vi "Mark10.vi"(0 "Requested Load":dbl, 1 "Data In":T1={"Message"="", "Homed?"=FALSE, "NextState"=enum."Timeout", "G.Load"=0.0, "G.Position"=0.0, "Load#"=0, "[G.Loads]"=[], "[TotalLoads]"=[], "[Errors]"=[], "ZeroWait"=0, "Results"=[], "DwellWait"=FALSE, "Test Result"=FALSE, "[CondyleLoads]"=[], "[Max]"=[], "[Min]"=[], "Valid String?"=FALSE, "ScanTime"=timestamp(0 s since 1904-01-01), "ScannedString"="", "LabelDevID"=0, "MfgDate"=timestamp(0 s since 1904-01-01), "[EEPROM Cmds]"=[], "[CalData]"=[], "[A/Ds]"=[], "[A/Dmax]"=[], "[A/Dmin]"=[], "BattMax"=0.0, "BattMin"=0.0, "DwellTime"=2000, "PendingDeviceType"="", "Zero G.load"=0.0, "GAINC Value"="", "Programming Step"=enum."Load EEPROM", "Front Panel Program?"=FALSE, "Final Program?"=FALSE, "PCB Score"=100, "AssyScore"=100, "Pass/Fail #"="", "Result String"="", "Programming Mode"=enum."Initial Program", "Angle Test Step"=enum."Initialize", "Accel Values"=[], "Shutdown Counter"=0, "V1"=0, "V2"=0, "V3"=0, "V4"=0, "EEPROM Data"=[], "Counter"=0, "Page#"=0, "Timer"=timestamp(0 s since 1904-01-01), "Use Mark10?"=FALSE, "Eng-Result#"=0, "DUT Serial #"=0, "Scroll Message?"=FALSE, "Clear Message"=FALSE, "Batt Test Step "=enum."Initialize", "RXTX Window Found?"=FALSE, "Shutdown First Call?"=FALSE, "A2 Delay (msec)"=500, "Support Script"={"Script #"="", "Script Revision"="", "[OEMs]"=[], "[[DeviceTypes]]"=[], "[[DeviceTypesVals]]"=[], "[[List of Errors]]"=[], "Default GAINC"="", "[[ASICtrims]]"=[], "ID For Echo"="", "Condyle A CalFactor"=100, "Condyle B CalFactor"=100, "[OEMs Prefix]"=[], "Packet ID 18"="", "[[Force Table Load Test]]"=[], "[[Force Table AccurTest]]"=[]}, "Serial Table"={"Serial File Path"=path "", "[[Serial Lookup Table]]"=[], "Serial Device Info"=[], "Valid Serial?"=FALSE}, "Target Information"={"Target Brand"="", "Target DeviceType"="", "Target Serial#"=100, "Target Lot#"=0, "Target DevID"=0, "Target Channel"=5}, "Operator"="", "COM Port"="", "Config Path"=path "", "Tx Array"=[], "DUT Parameters"={"Channel"=0, "DeviceID"=0, "Script Rev"=0, "Month"=0, "Day"=0, "Year"=0, "Lot#"=0, "V1"=0, "V2"=0, "V3"=0, "V4"=0, "MFG"=0, "Cal FactorA 10"=0, "Cal FactorB 10  "=0, "Cal FactorA 16"=0, "Cal FactorB 16"=0, "ASICtrim"=[], "TmpChan"=0, "GAINC"="", "Brand"="", "Device"="", "Serial #"=0, "Batt310"=0, "Batt 280"=0}, "FTS Main?"=FALSE, "Loading"={"[Forces]"=[], "[Dwell]"=[], "Loading Step"=enum."Initialize Test"}, "Software Version"="", "Correction Factor"="", "Second Load Test"=FALSE, "Acc Loads"=[], "Mark10 Config"={"H2S%"=[80.0, 85.0, 90.0, 95.0, 100.0], "H2S Speed"=[12.0, 8.0, 6.0, 4.0, 2.0], "H to S"=2.0, "Home Speed"=1.0, "LoadWin"=0.0, "Load Speed"=0.0, "PID"={"Kp"=0.04, "Kd"=0.005001, "Ki"=2.9999999999999923e-05}}, "Channels"={"Transceiver Ch"=5, "Operating Ch"=5, "Start Ch"=0}, "Channel EEPROM"=[], "Load Notes"=[], "Engr Log?"=FALSE, "Time"=[], "Program Retry"=FALSE, "Operator Channel"="", "Target Channel "="", "New Data Program"=FALSE, "NFHU Pass?"=FALSE, "Cycle Number"=0, "Cal Cycle#"=0, "[Avg G.Loads] "=[], "[Avg A/Ds] "=[], "Cal Retry?"=FALSE, "[Total A/Ds]  "=[], "Cycle Num LA"=0, "LA Cycle# "=0, "Shim Num"=0, "Shim#  "=0, "Angle Test?"=FALSE} {"Mark10 Config"."PID"."Ki" min=0.0 max=200.0 format="%.6f"; "Mark10 Config"."PID"."Kd" min=0.0 max=200.0 format="%.6f"; "Mark10 Config"."PID"."Kp" min=0.0 max=200.0 format="%.6f"; "DUT Parameters"."ASICtrim" format="%02x"}, 2 "Stop?":bool, 3 "Requested Position":dbl, 4 "Accuracy \nTest?":bool, 5 "error in (no error)":errorcluster, 9 "Action":T16=enum."Stop Motor") -> (10 "Flags":T15, 14 "Live Load":dbl, 16 "Live Position":dbl, 17 "Done?":bool, 19 "error out":errorcluster)   [LabVIEW 2015]
uses:
  Controls/Mark10 states.ctl
  Controls/LocalVars.ctl
  Controls/Gen2 FT states.ctl
  Controls/Iniial Device Programming.ctl
  SubVI/ProgramStageControl.ctl
  Controls/Batt Cap Steps.ctl
  Controls/Support Script.ctl
  Controls/Serial Table.ctl
  Controls/Device Information.ctl
  Controls/InfoPacket.ctl
  Controls/Loading.ctl
  Controls/Load Step.ctl
  Controls/Mark10 Config.ctl
  Controls/PID parameters.ctl
  Controls/Channels.ctl
  Controls/Mark10.ctl
  Controls/Mark10 Comm states.ctl
panel:
  in  "Speed":dbl
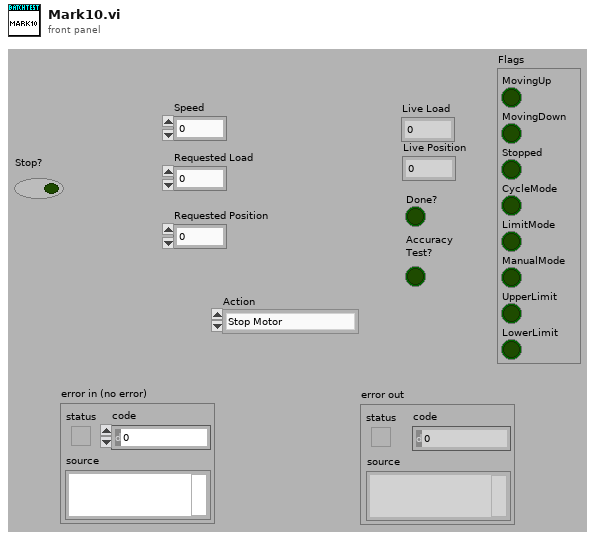
[diagram p1: front panel]
types:
  T1 = typedef "LocalVars.ctl" = cluster{"Message":string, "Homed?":bool, "NextState":T2, "G.Load":dbl, "G.Position":dbl, "Load#":i32, "[G.Loads]":dbl[], "[TotalLoads]":dbl[], "[Errors]":dbl[][], "ZeroWait":u32, "Results":dbl[], "DwellWait":bool, "Test Result":bool, "[CondyleLoads]":dbl[][], "[Max]":dbl[], "[Min]":dbl[], "Valid String?":bool, "ScanTime":timestamp, "ScannedString":string, "LabelDevID":u32, "MfgDate":timestamp, "[EEPROM Cmds]":u8[][], "[CalData]":u8[][], "[A/Ds]":dbl[][], "[A/Dmax]":dbl[], "[A/Dmin]":dbl[], "BattMax":dbl, "BattMin":dbl, "DwellTime":i32, "PendingDeviceType":string, "Zero G.load":dbl, "GAINC Value":string, "Programming Step":T3, "Front Panel Program?":bool, "Final Program?":bool, "PCB Score":i32, "AssyScore":i32, "Pass/Fail #":string, "Result String":string, "Programming Mode":T4, "Angle Test Step":enum16{"Initialize", "Get X", "Get Y", "Get Z", "Next Test"}, "Accel Values":dbl[][], "Shutdown Counter":u32, "V1":i32, "V2":i32, "V3":i32, "V4":i32, "EEPROM Data":i32[][], "Counter":i32, "Page#":i32, "Timer":timestamp, "Use Mark10?":bool, "Eng-Result#":u32, "DUT Serial #":i32, "Scroll Message?":bool, "Clear Message":bool, "Batt Test Step ":T5, "RXTX Window Found?":bool, "Shutdown First Call?":bool, "A2 Delay (msec)":i16, "Support Script":T6, "Serial Table":T7, "Target Information":T8, "Operator":string, "COM Port":string, "Config Path":path, "Tx Array":u8[], "DUT Parameters":T9, "FTS Main?":bool, "Loading":T10, "Software Version":string, "Correction Factor":string, "Second Load Test":bool, "Acc Loads":dbl[][], "Mark10 Config":T12, "Channels":T14, "Channel EEPROM":i32[][], "Load Notes":string[], "Engr Log?":bool, "Time":timestamp[], "Program Retry":bool, "Operator Channel":string, "Target Channel ":string, "New Data Program":bool, "NFHU Pass?":bool, "Cycle Number":i32, "Cal Cycle#":i32, "[Avg G.Loads] ":dbl[], "[Avg A/Ds] ":dbl[][], "Cal Retry?":bool, "[Total A/Ds]  ":dbl[][], "Cycle Num LA":i32, "LA Cycle# ":i32, "Shim Num":i32, "Shim#  ":i32, "Angle Test?":bool}
  T2 = typedef "Gen2 FT states.ctl" = enum16{"---------SETUP-------", "Initialization", "Read Support Data", "Initialize Mark-10", "Initialize Transceiver", "------UTILITIES------", "Change DUT Channel", "Find RxTx Window", "Reset Device", "Scan Channels", "Read Serial Lookup", "Shutdown Device", "ESTOP", "--------USER---------", "Timeout", "-----PROGRAM-----", "Program Device", "------MARK10--------", "Go Home", "MoveUp", "MoveDown", "Goto Load", "Goto Position", "Stop Motor", "---------TESTS--------", "Start Test", "Angle Test", "Load Test", "Load Accuracy Test", "Battery Test", "------RESULTS-------", "End Test", "Display Result", "--------EXIT--------", "Exit"}
  T3 = typedef "Iniial Device Programming.ctl" = enum16{"Load EEPROM", "Send First A1", "Send EEPROM", "Send A1", "Check EEPROM Echo", "Verify transmission", "Programming Successful", "Programming Failed"}
  T4 = typedef "ProgramStageControl.ctl" = enum16{"Initial Program", "GainC", "Scales"}
  T5 = typedef "Batt Cap Steps.ctl" = enum16{"Initialize", "Collect 2.8 Volts", "Collect 3.1 Volts", "Check Results"}
  T6 = typedef "Support Script.ctl" = cluster{"Script #":string, "Script Revision":string, "[OEMs]":string[], "[[DeviceTypes]]":string[][], "[[DeviceTypesVals]]":u16[][], "[[List of Errors]]":string[][], "Default GAINC":string, "[[ASICtrims]]":u8[][], "ID For Echo":string, "Condyle A CalFactor":i32, "Condyle B CalFactor":i32, "[OEMs Prefix]":string[], "Packet ID 18":string, "[[Force Table Load Test]]":dbl[][], "[[Force Table AccurTest]]":dbl[][]}
  T7 = typedef "Serial Table.ctl" = cluster{"Serial File Path":path, "[[Serial Lookup Table]]":string[][], "Serial Device Info":string[], "Valid Serial?":bool}
  T8 = typedef "Device Information.ctl" = cluster{"Target Brand":string, "Target DeviceType":string, "Target Serial#":i32, "Target Lot#":u32, "Target DevID":u32, "Target Channel":u8}
  T9 = typedef "InfoPacket.ctl" = cluster{"Channel":u8, "DeviceID":u32, "Script Rev":u8, "Month":u8, "Day":u8, "Year":u8, "Lot#":u32, "V1":u16, "V2":u16, "V3":u16, "V4":u16, "MFG":u8, "Cal FactorA 10":u8, "Cal FactorB 10  ":u8, "Cal FactorA 16":u8, "Cal FactorB 16":u8, "ASICtrim":u8[], "TmpChan":u8, "GAINC":string, "Brand":string, "Device":string, "Serial #":u64, "Batt310":u16, "Batt 280":u16}
  T10 = typedef "Loading.ctl" = cluster{"[Forces]":dbl[], "[Dwell]":dbl[], "Loading Step":T11}
  T11 = typedef "Load Step.ctl" = enum16{"Initialize Test", "Go Home", "Detect Dev Surface", "Wait to zero Device", "Zero Device", "Do Test", "Test Result"}
  T12 = typedef "Mark10 Config.ctl" = cluster{"H2S%":dbl[], "H2S Speed":dbl[], "H to S":dbl, "Home Speed":dbl, "LoadWin":dbl, "Load Speed":dbl, "PID":T13}
  T13 = typedef "PID parameters.ctl" = cluster{"Kp":dbl, "Kd":dbl, "Ki":dbl}
  T14 = typedef "Channels.ctl" = cluster{"Transceiver Ch":u8, "Operating Ch":u8, "Start Ch":u8}
  T15 = cluster{"MovingUp":bool, "MovingDown":bool, "Stopped":bool, "CycleMode":bool, "LimitMode":bool, "ManualMode":bool, "UpperLimit":bool, "LowerLimit":bool}
  T16 = typedef "Mark10 states.ctl" = enum16{"Initialize", "Go Home", "Move Up", "Move Down", "Stop @ Load", "Read Status", "Goto Position", "Goto Device Surface", "Stop Motor", "Shutdown", "Exit"}
  T17 = typedef "Mark10 Comm states.ctl" = enum16{"Open Session", "Get Reference", "Write Data", "Read Data", "Close Session"}
  T18 = typedef "Mark10.ctl" = cluster{"Mark10 Ref":refnum<visa-resource-name>, "Counter":i32, "MotorSpeed":dbl, "LastSpeed":dbl, "Live Load":dbl, "Live Position":dbl, "Stage":i32, "Speeds":dbl[], "DevFound?":bool, "DevPosition":dbl, "Flags":cluster{"MovingUp":bool, "MovingDown":bool, "Stopped":bool, "CycleMode":bool, "LimitMode":bool, "ManualMode":bool, "UpperLimit":bool, "LowerLimit":bool}, "Stopped?":bool, "ofPass":i32, "LastDrive":dbl, "Mark10 Config":T12}
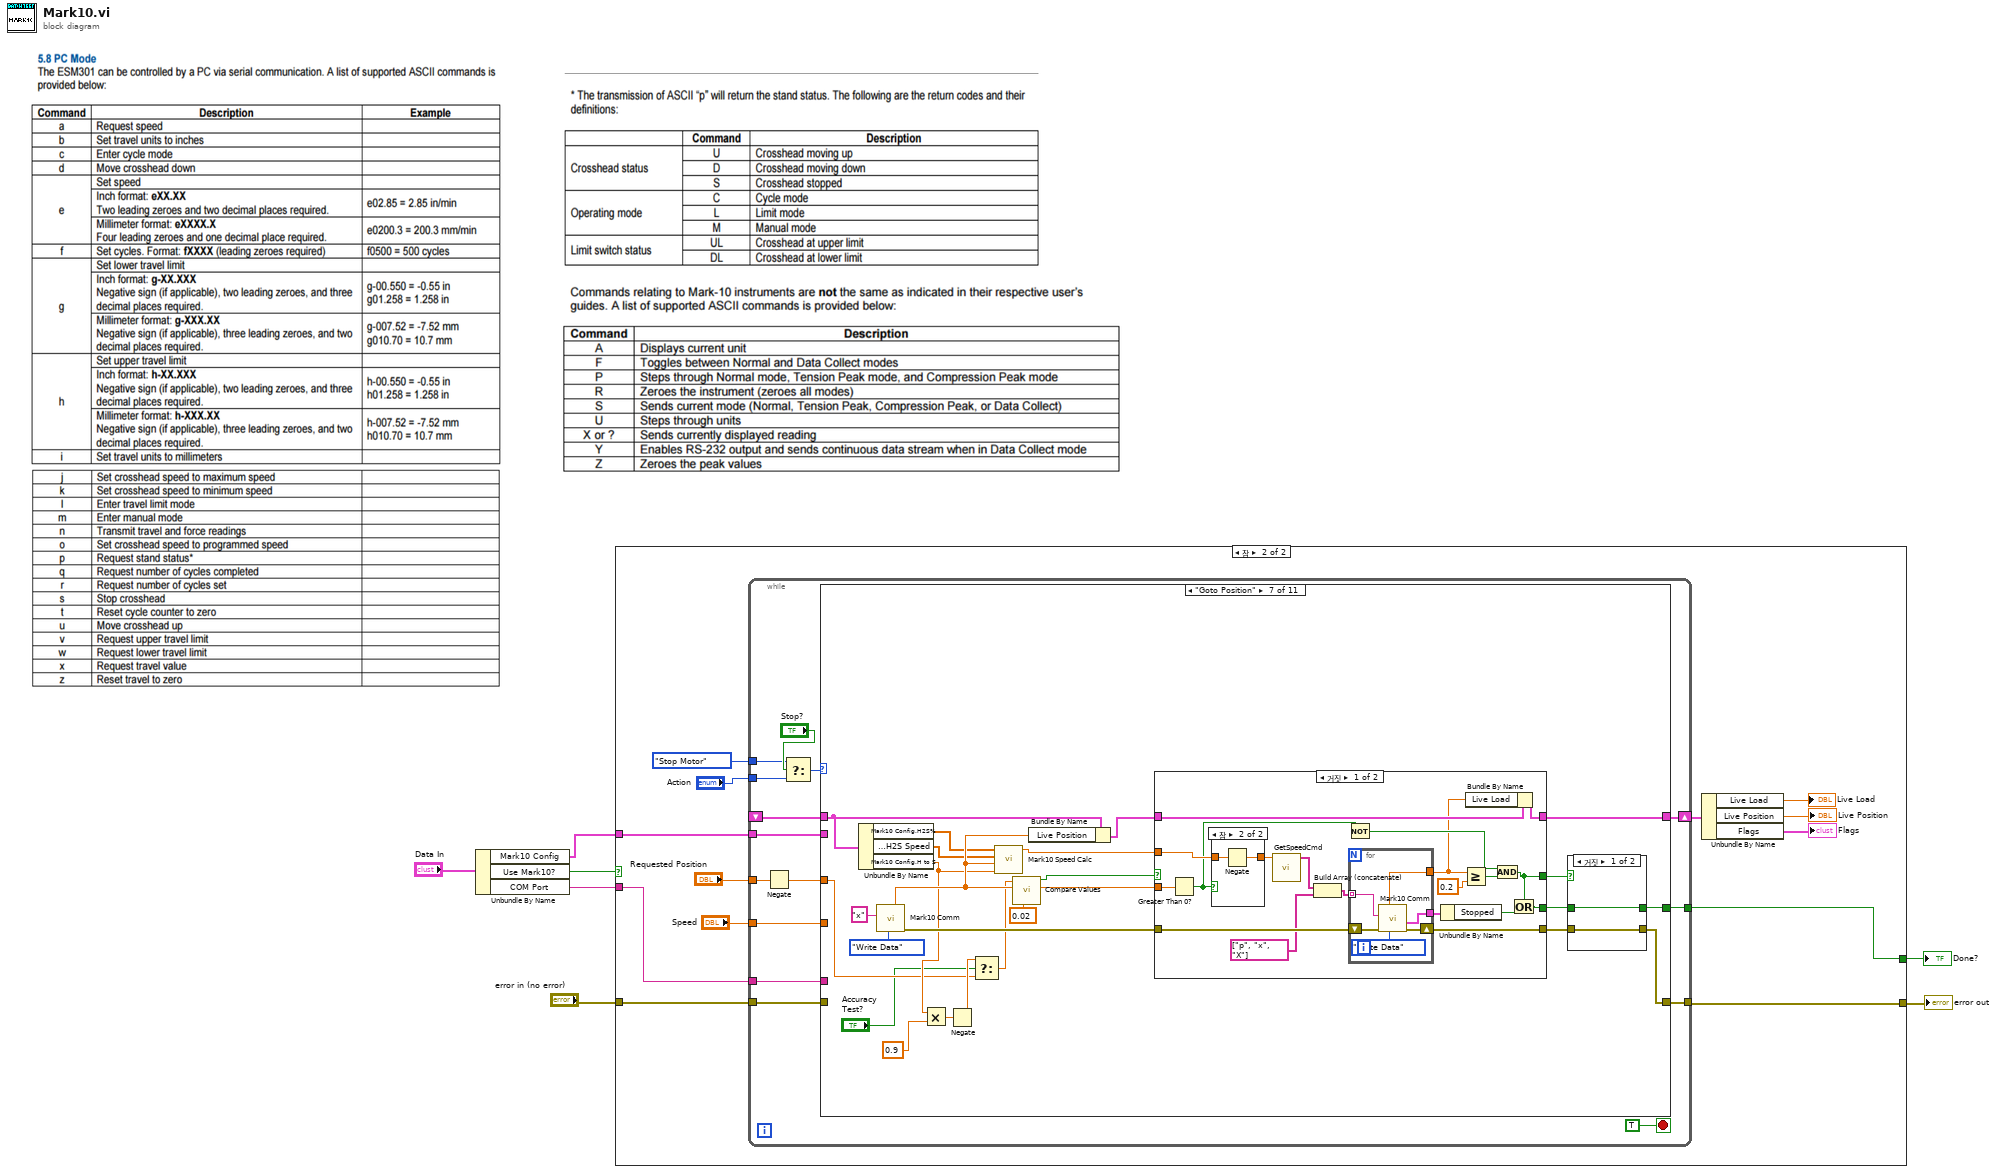
[diagram p0: block diagram]
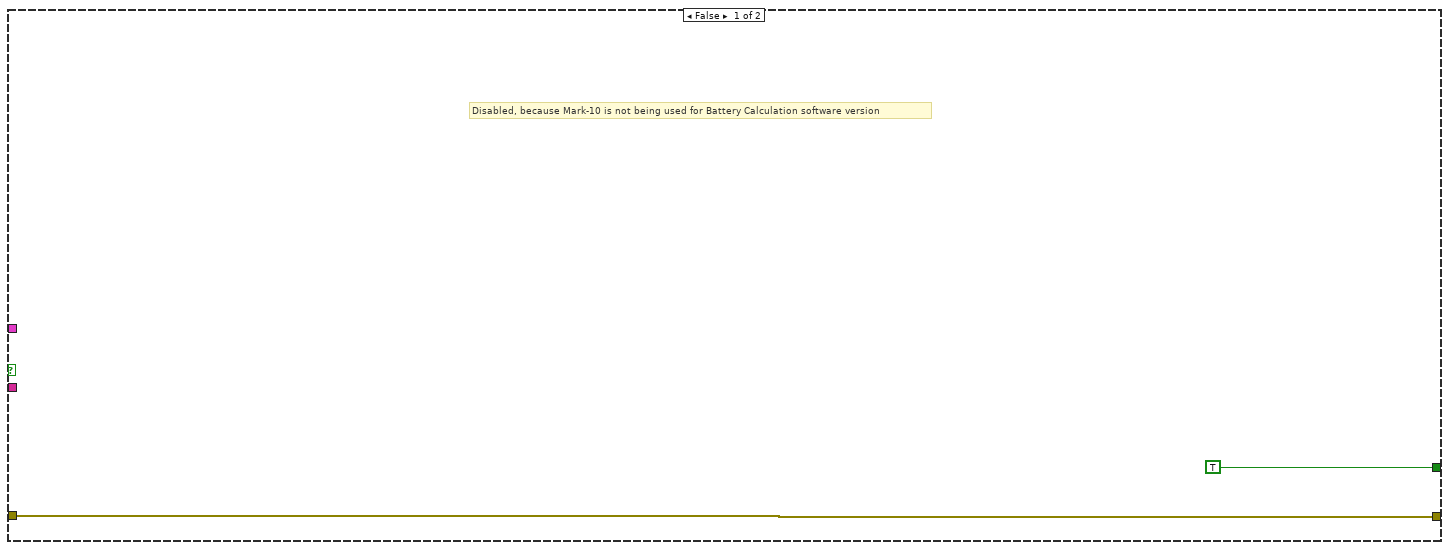
[diagram p2: hidden frame]
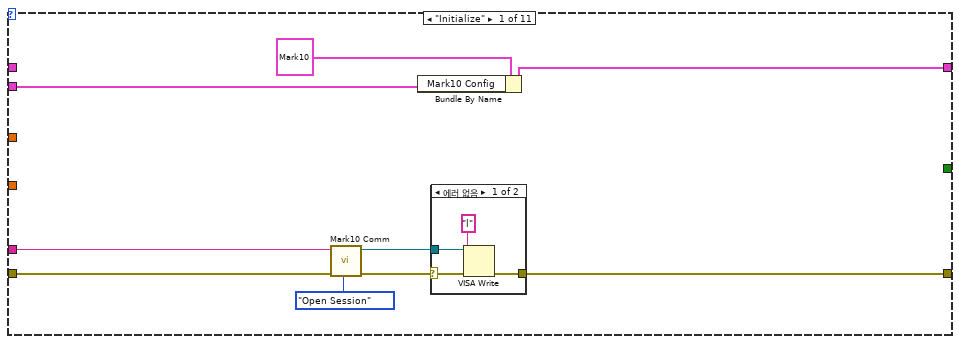
[diagram p3: hidden frame]
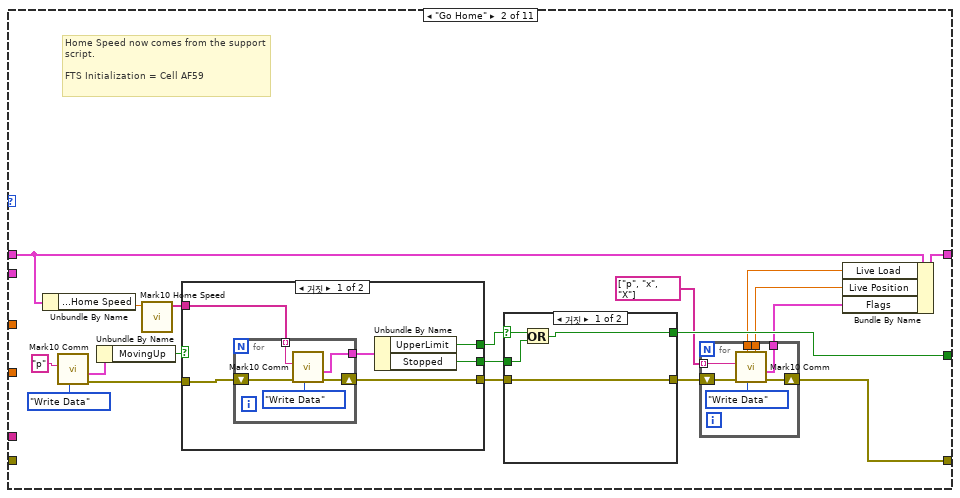
[diagram p5: hidden frame]
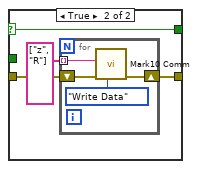
[diagram p6: hidden frame]
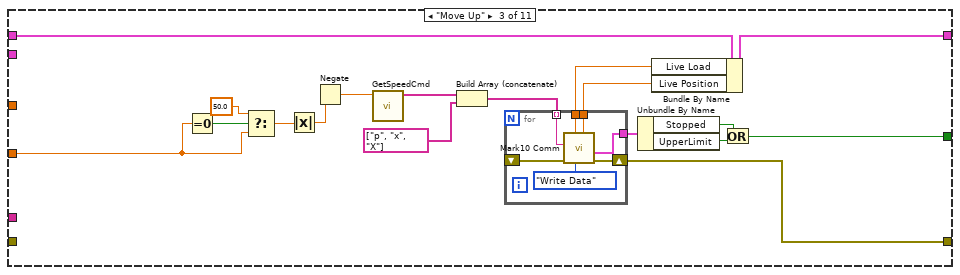
[diagram p8: hidden frame]
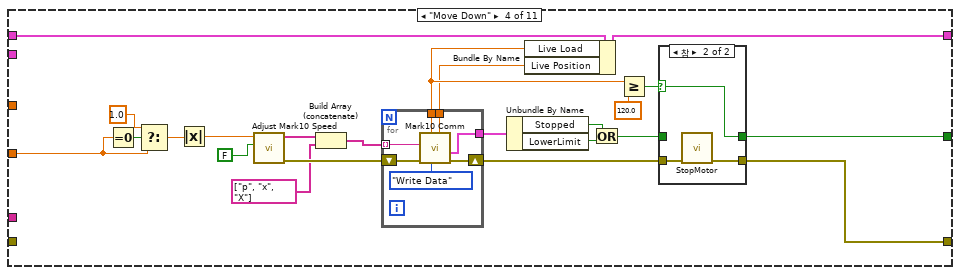
[diagram p9: hidden frame]
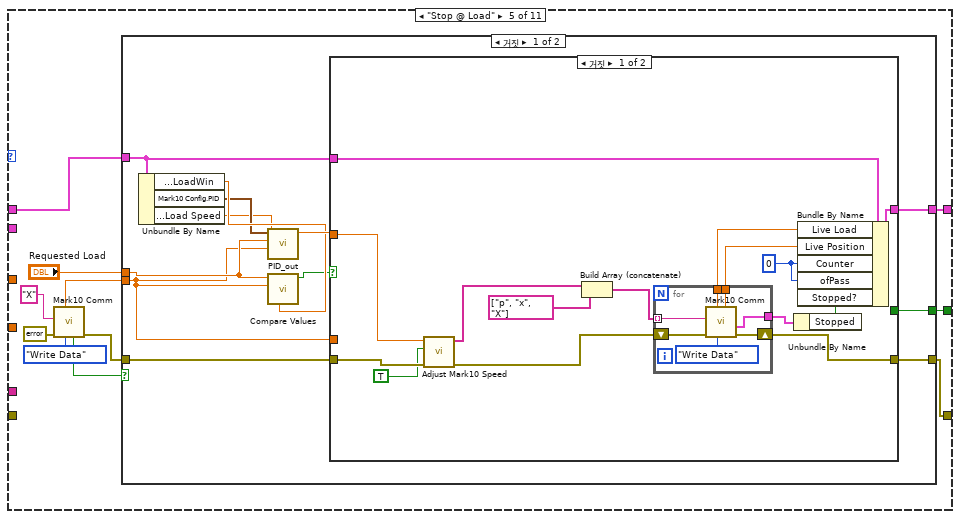
[diagram p11: hidden frame]
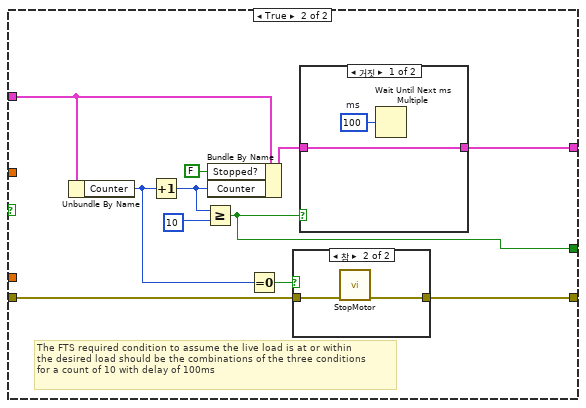
[diagram p12: hidden frame]
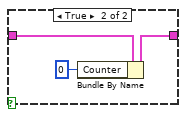
[diagram p14: hidden frame]
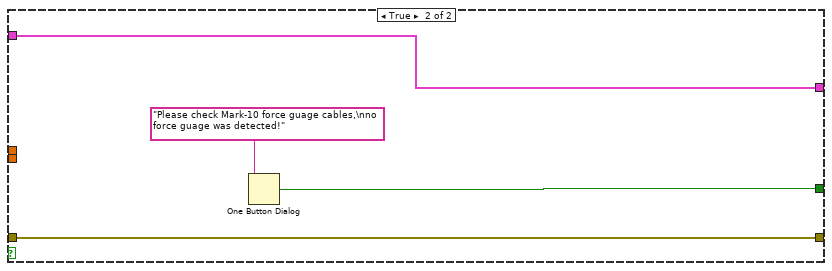
[diagram p15: hidden frame]
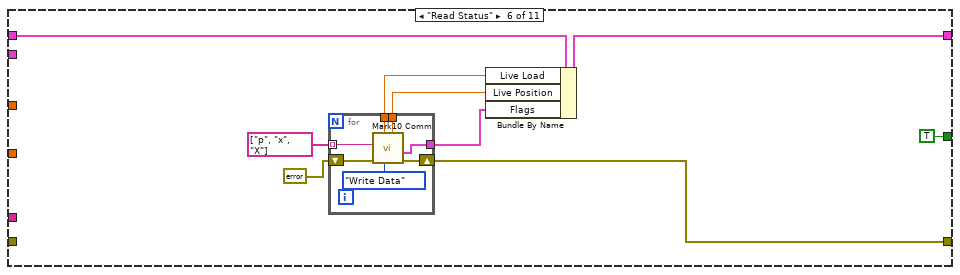
[diagram p16: hidden frame]
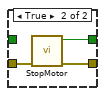
[diagram p17: hidden frame]
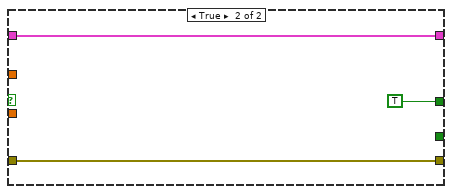
[diagram p19: hidden frame]
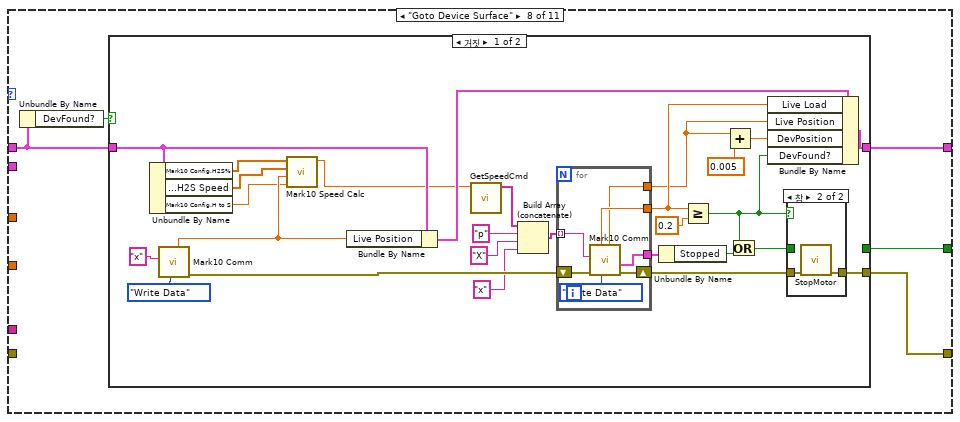
[diagram p20: hidden frame]
diagram:
  n1 = Unbundle By Name("Data In") -> ("Mark10 Config"=w2:T12, "Use Mark10?"=w6:bool, "COM Port"=w1:string)
  n2 = case shown="참" w6 {
    tunnel: "error in (no error)" -> [w9 w19]
    tunnel: [w9 w18] -> w4
    tunnel: [TRUE ("Stopped") w17] -> w3
    tunnel: w2 -> [_ w11]
    tunnel: w1 -> [_ w10]
    frame False {
      # "Disabled, because Mark-10 is not being used for Battery Calculation software version"
    }
    frame True {
      n3 = while {
        shift-right: [w36] -> w14
        shift-left: _ -> [w35]
        tunnel: [w37] -> w18
        tunnel: [w33] -> w17
        tunnel: Mark10_states."Stop Motor" ("t") -> [w30]
        tunnel: "Speed" -> [w29]
        tunnel: "Requested Position" -> [w28]
        tunnel: "Action" -> [w27]
        tunnel: w10 -> [w25]
        tunnel: w19 -> [w24]
        tunnel: w11 -> [w23]
        stop <- TRUE stop-if-true
        n4 = Negate(x=w28) -> (-x=w26:dbl)
        n5 = Select(t=w30, s="Stop?", f=w27) -> (s? t:f=w31:T16)
        n6 = case shown="\"Goto Position\"" w31 {
          tunnel: [w44 w60 w119 w134 w166 w237 w263 w310 w385 _ w388] -> w37
          tunnel: [w39 w58 w104 w131 w163 w236 w259 w311 w383 w387 w390] -> w36
          tunnel: w35 -> [_ w52 w113 w145 w162 w238 w256 w308 w386 w387 w390]
          tunnel: [_ w64 w118 w132 w164 TRUE ("Stopped") w261 w309 w384 _ _] -> w33
          tunnel: w29 -> [_ _ w115 w147 _ _ _ _ _ _ _]
          tunnel: w26 -> [_ _ _ _ _ _ w247 _ _ _ _]
          tunnel: w25 -> [w41 _ _ _ _ _ _ _ _ _ _]
          tunnel: w24 -> [w40 _ _ _ _ _ _ _ _ _ _]
          tunnel: w23 -> [w38 _ _ _ _ _ _ _ _ _ _]
          frame "Initialize" {
            n7 = call "Mark10 Comm.vi"("Action"=Mark10_Comm_states."Open Session", "error in (no error)"=w40, "VISA resource name"=w41) -> ("error out"=w45:errorcluster, "Mark-10 Ref"=w43:refnum<visa-resource-name>)  [unwired: 2 in, 5 out]
            n8 = Bundle By Name(cluster=T18 {"Mark10 Ref"="", "Counter"=0, "MotorSpeed"=0.0, "LastSpeed"=0.0, "Live Load"=0.0, "Live Position"=0.0, "Stage"=0, "Speeds"=[], "DevFound?"=FALSE, "DevPosition"=0.0, "Flags"={"MovingUp"=FALSE, "MovingDown"=FALSE, "Stopped"=FALSE, "CycleMode"=FALSE, "LimitMode"=FALSE, "ManualMode"=FALSE, "UpperLimit"=FALSE, "LowerLimit"=FALSE}, "Stopped?"=FALSE, "ofPass"=0, "LastDrive"=0.0, "Mark10 Config"={"H2S%"=[], "H2S Speed"=[], "H to S"=0.0, "Home Speed"=0.0, "LoadWin"=0.0, "Load Speed"=0.0, "PID"={"Kp"=0.0, "Kd"=0.0, "Ki"=0.0}}}, "Mark10 Config"=w38) -> (w39:T18)
            n9 = case shown="에러 없음" w45 {
              selector: w45 -> [w49 w51]
              tunnel: w43 -> [w50 _]
              tunnel: [w48 w51] -> w44
              frame No Error {
                n10 = VISA Write(VISA resource name=w50, write buffer="l", error in (no error)=w49) -> (error out=w48:errorcluster)  [unwired: 2 out]
              }
              frame Error {
              }
            }
          }
          frame "Go Home" {
            # "Home Speed now comes from the support script. \n\nFTS Initialization = Cell AF59"
            n11 = Unbundle By Name(w52) -> ("Mark10 Config.Home Speed"=w54:dbl)
            n12 = call "Mark10 Comm.vi"("Action"=Mark10_Comm_states."Write Data", "Write"="p") -> ("error out"=w66:errorcluster, "Flags"=w68:T15)  [unwired: 3 in, 5 out]
            n13 = Unbundle By Name(w68) -> ("MovingUp"=w67:bool)
            n14 = call "Mark10 Home Speed.vi"("Speed"=w54) -> ("Cmds"=w53:string[])  [unwired: 10 in]
            n15 = case shown="거짓" w67 {
              tunnel: w66 -> [w95 w101]
              tunnel: [w94 w101] -> w65
              tunnel: [w92 _] -> w63
              tunnel: [w91 _] -> w62
              tunnel: w53 -> [w90 _]
              frame False {
                n16 = for {
                  tunnel: w90 -> [w99] mode=indexing
                  shift-right: [w98] -> w94
                  shift-left: w95 -> [w97]
                  tunnel: [w96] -> w93
                  n17 = call "Mark10 Comm.vi"("Action"=Mark10_Comm_states."Write Data", "error in (no error)"=w97, "Write"=w99) -> ("error out"=w98:errorcluster, "Flags"=w96:T15)  [unwired: 2 in, 5 out]
                }
                n18 = Unbundle By Name(w93) -> ("UpperLimit"=w92:bool, "Stopped"=w91:bool)
              }
              frame True {
              }
            }
            n19 = case shown="거짓" w63 {
              selector: w63 -> [w80 w85]
              tunnel: w65 -> [w81 w82]
              tunnel: [w81 w83] -> w61
              tunnel: [w78 w85] -> w64
              tunnel: w62 -> [w79 _]
              frame False {
                n20 = Or(x=w80, y=w79) -> (x .or. y?=w78:bool)
              }
              frame True {
                n21 = for {
                  shift-right: [w88] -> w83
                  shift-left: w82 -> [w87]
                  tunnel: string[] ["z", "R"] -> [w86] mode=indexing
                  n22 = call "Mark10 Comm.vi"("Action"=Mark10_Comm_states."Write Data", "error in (no error)"=w87, "Write"=w86) -> ("error out"=w88:errorcluster)  [unwired: 2 in, 6 out]
                }
              }
            }
            n23 = for {
              shift-right: [w76] -> w60
              shift-left: w61 -> [w75]
              tunnel: string[] ["p", "x", "X"] -> [w74] mode=indexing
              tunnel: [w73] -> w57
              tunnel: [w72] -> w56
              tunnel: [w71] -> w55
              n24 = call "Mark10 Comm.vi"("Action"=Mark10_Comm_states."Write Data", "error in (no error)"=w75, "Write"=w74) -> ("error out"=w76:errorcluster, "Flags"=w73:T15, "Position"=w72:dbl, "Load"=w71:dbl)  [unwired: 2 in, 3 out]
            }
            n25 = Bundle By Name(cluster=w52, "Live Load"=w55, "Live Position"=w56, "Flags"=w57) -> (w58:T18)
          }
          frame "Move Up" {
            n26 = Equal To 0?(x=w115) -> (x = 0?=w117:bool)
            n27 = Select(t=50.0, s=w117, f=w115) -> (s? t:f=w114:dbl)
            n28 = Absolute Value(x=w114) -> (abs(x)=w107:dbl)
            n29 = Negate(x=w107) -> (-x=w108:dbl)
            n30 = call "GetSpeedCmd.vi"("Speed"=w108) -> ("Cmds"=w110:string[])  [unwired: 10 in]
            n31 = Build Array (concatenate)(w110, string[] ["p", "x", "X"]) -> (w109:string[])
            n32 = for {
              tunnel: w109 -> [w125] mode=indexing
              shift-right: [w124] -> w119
              shift-left: _ -> [w123]
              tunnel: [w122] -> w111
              tunnel: [w121] -> w103
              tunnel: [w120] -> w102
              n33 = call "Mark10 Comm.vi"("Action"=Mark10_Comm_states."Write Data", "error in (no error)"=w123, "Write"=w125) -> ("error out"=w124:errorcluster, "Flags"=w122:T15, "Position"=w120:dbl, "Load"=w121:dbl)  [unwired: 2 in, 3 out]
            }
            n34 = Unbundle By Name(w111) -> ("Stopped"=w106:bool, "UpperLimit"=w112:bool)
            n35 = Bundle By Name(cluster=w113, "Live Load"=w103, "Live Position"=w102) -> (w104:T18)
            n36 = Or(x=w106, y=w112) -> (x .or. y?=w118:bool)
          }
          frame "Move Down" {
            n37 = Equal To 0?(x=w147) -> (x = 0?=w149:bool)
            n38 = Select(t=1.0, s=w149, f=w147) -> (s? t:f=w146:dbl)
            n39 = Absolute Value(x=w146) -> (abs(x)=w140:dbl)
            n40 = call "Adjust Mark10 Speed.vi"("load test?"=FALSE, "Requested Speed"=w140) -> ("error out"=w139:errorcluster, "Cmds"=w138:string[])  [unwired: 8 in]
            n41 = Build Array (concatenate)(w138, string[] ["p", "x", "X"]) -> (w142:string[])
            n42 = for {
              tunnel: w142 -> [w160] mode=indexing
              shift-right: [w159] -> w135
              shift-left: w139 -> [w158]
              tunnel: [w157] -> w143
              tunnel: [w156] -> w129
              tunnel: [w155] -> w128
              n43 = call "Mark10 Comm.vi"("Action"=Mark10_Comm_states."Write Data", "error in (no error)"=w158, "Write"=w160) -> ("error out"=w159:errorcluster, "Flags"=w157:T15, "Position"=w155:dbl, "Load"=w156:dbl)  [unwired: 2 in, 3 out]
            }
            n44 = Unbundle By Name(w143) -> ("Stopped"=w141:bool, "LowerLimit"=w144:bool)
            n45 = Bundle By Name(cluster=w145, "Live Load"=w129, "Live Position"=w128) -> (w131:T18)
            n46 = Or(x=w141, y=w144) -> (x .or. y?=w133:bool)
            n47 = Greater Or Equal?(x=w129, y=120.0) -> (x >= y?=w136:bool)
            n48 = case shown="참" w136 {
              selector: w136 -> [_ w152]
              tunnel: w135 -> [w151 w154]
              tunnel: [w151 w153] -> w134
              tunnel: [w150 w152] -> w132
              tunnel: w133 -> [w150 _]
              frame False {
              }
              frame True {
                n49 = call "StopMotor.vi"("error in (no error)"=w154) -> ("error out"=w153:errorcluster)  [unwired: 9 in, 1 out]
              }
            }
          }
          frame "Stop @ Load" {
            n50 = call "Mark10 Comm.vi"("Action"=Mark10_Comm_states."Write Data", "error in (no error)"=errorcluster {"status"=FALSE, "code"=0, "source"=""} ("error out"), "Write"="X") -> ("error out"=w167:errorcluster, "NoGauge"=w165:bool, "Load"=w170:dbl)  [unwired: 2 in, 4 out]
            n51 = case shown="거짓" w165 {
              tunnel: "Requested Load" -> [w180 _]
              tunnel: w170 -> [w179 _]
              tunnel: w167 -> [w184 w227]
              tunnel: [w183 w227] -> w166
              tunnel: [w182 w228] -> w164
              tunnel: [w181 w226] -> w163
              tunnel: w162 -> [w177 w226]
              frame False {
                n52 = Unbundle By Name(w177) -> ("Mark10 Config.LoadWin"=w176:dbl, "Mark10 Config.PID"=w175:T13, "Mark10 Config.Load Speed"=w174:dbl)
                n53 = call "PID_out.vi"("Load Speed"=w174, "Live Load"=w179, "Target Load"=w180, "PID"=w175) -> ("Out Speed"=w178:dbl)  [unwired: 6 in, 1 out]
                n54 = call "Compare Values.vi"("Compare Window"=w176, "Value2 In"=w179, "Value1 In"=w180) -> ("Within Window?"=w173:bool)  [unwired: 7 in, 1 out]
                n55 = case shown="거짓" w173 {
                  tunnel: w184 -> [w195 w216]
                  tunnel: [w199 w215] -> w183
                  tunnel: [_ w210] -> w182
                  tunnel: [w198 w217] -> w181
                  tunnel: w177 -> [w186 w214]
                  tunnel: w179 -> [_ _]
                  tunnel: w178 -> [w187 _]
                  frame False {
                    w188 = 0 ("Counter")
                    n56 = call "Adjust Mark10 Speed.vi"("error in (no error)"=w195, "load test?"=TRUE, "Requested Speed"=w187) -> ("error out"=w194:errorcluster, "Cmds"=w197:string[])  [unwired: 7 in]
                    n57 = Build Array (concatenate)(w197, string[] ["p", "x", "X"]) -> (w196:string[])
                    n58 = for {
                      tunnel: w196 -> [w205] mode=indexing
                      shift-right: [w204] -> w199
                      shift-left: w194 -> [w203]
                      tunnel: [w202] -> w193
                      tunnel: [w201] -> w191
                      tunnel: [w200] -> w190
                      n59 = call "Mark10 Comm.vi"("Action"=Mark10_Comm_states."Write Data", "error in (no error)"=w203, "Write"=w205) -> ("error out"=w204:errorcluster, "Flags"=w202:T15, "Position"=w201:dbl, "Load"=w200:dbl)  [unwired: 2 in, 3 out]
                    }
                    n60 = Unbundle By Name(w193) -> ("Stopped"=w192:bool)
                    n61 = Bundle By Name(cluster=w186, "Live Load"=w190, "Live Position"=w191, "Counter"=w188, "ofPass"=w188, "Stopped?"=w192) -> (w198:T18)
                  }
                  frame True {
                    # "The FTS required condition to assume the live load is at or within\nthe desired load should be the combinations of the three conditions\nfor a count of 10 with delay of 100ms"
                    n62 = Unbundle By Name(w214) -> ("Counter"=w208:i32)
                    n63 = Increment(x=w208) -> (x+1=w209:i32)
                    n64 = Greater Or Equal?(x=w209, y=10) -> (x >= y?=w210:bool)
                    n65 = Bundle By Name(cluster=w214, "Stopped?"=FALSE, "Counter"=w209) -> (w213:T18)
                    n66 = Equal To 0?(x=w208) -> (x = 0?=w207:bool)
                    n67 = case shown="참" w207 {
                      tunnel: w216 -> [w218 w220]
                      tunnel: [w218 w219] -> w215
                      frame False {
                      }
                      frame True {
                        n68 = call "StopMotor.vi"("error in (no error)"=w220) -> ("error out"=w219:errorcluster)  [unwired: 9 in, 1 out]
                      }
                    }
                    n69 = case shown="거짓" w210 {
                      tunnel: [w222 w224] -> w217
                      tunnel: w213 -> [w222 w225]
                      frame False {
                        w221 = u32 100  # ms
                        n70 = Wait Until Next ms Multiple(millisecond multiple=w221) -> ()  [unwired: 1 out]
                      }
                      frame True {
                        n71 = Bundle By Name(cluster=w225, "Counter"=0) -> (w224:T18)
                      }
                    }
                  }
                }
              }
              frame True {
                n72 = One Button Dialog(message="Please check Mark-10 force guage cables,\nno force guage was detected!") -> (true=w228:bool)  [unwired: 1 in]
              }
            }
          }
          frame "Read Status" {
            n73 = for {
              tunnel: [w243] -> w235
              tunnel: string[] ["p", "x", "X"] -> [w242] mode=indexing
              shift-right: [w244] -> w237
              shift-left: errorcluster {"status"=FALSE, "code"=0, "source"=""} ("error out") -> [w241]
              tunnel: [w240] -> w232
              tunnel: [w239] -> w231
              n74 = call "Mark10 Comm.vi"("Action"=Mark10_Comm_states."Write Data", "error in (no error)"=w241, "Write"=w242) -> ("error out"=w244:errorcluster, "Flags"=w239:T15, "Position"=w240:dbl, "Load"=w243:dbl)  [unwired: 2 in, 3 out]
            }
            n75 = Bundle By Name(cluster=w238, "Live Load"=w235, "Live Position"=w232, "Flags"=w231) -> (w236:T18)
          }
          frame "Goto Position" {
            n76 = Unbundle By Name(w256) -> ("Mark10 Config.H2S%"=w254:dbl[], "Mark10 Config.H2S Speed"=w253:dbl[], "Mark10 Config.H to S"=w250:dbl)
            n77 = call "Mark10 Comm.vi"("Action"=Mark10_Comm_states."Write Data", "Write"="x" ("element")) -> ("error out"=w267:errorcluster, "Position"=w255:dbl)  [unwired: 3 in, 5 out]
            n78 = Multiply(x=w250, y=0.9) -> (x*y=w251:dbl)
            n79 = Negate(x=w251) -> (-x=w249:dbl)
            n80 = Select(t=w249, s="Accuracy \nTest?", f=w247) -> (s? t:f=w248:dbl)
            n81 = call "Mark10 Speed Calc.vi"("Home to Surface"=w250, "Live Position"=w255, "H2S Speed"=w253, "H2S %"=w254) -> ("Speed Output"=w257:dbl)  [unwired: 7 in]
            n82 = call "Compare Values.vi"("Compare Window"=0.02, "Value2 In"=w255, "Value1 In"=w248) -> ("Delta Out"=w265:dbl, "Within Window?"=w266:bool)  [unwired: 7 in]
            n83 = Bundle By Name(cluster=w256, "Live Position"=w255) -> (w258:T18)
            n84 = case shown="거짓" w266 {
              tunnel: w267 -> [w294 w305]
              tunnel: [w293 w305] -> w264
              tunnel: [w286 _] -> w260
              tunnel: w265 -> [w292 _]
              tunnel: w257 -> [w285 _]
              tunnel: [w282 TRUE] -> w262
              tunnel: [w277 w304] -> w259
              tunnel: w258 -> [w278 w304]
              frame False {
                n85 = Greater Than 0?(x=w292) -> (x > 0?=w281:bool)
                n86 = case shown="참" w281 {
                  tunnel: w285 -> [w295 w297]
                  tunnel: [w295 w296] -> w284
                  frame False {
                  }
                  frame True {
                    n87 = Negate(x=w297) -> (-x=w296:dbl)
                  }
                }
                n88 = call "GetSpeedCmd.vi"("Speed"=w284) -> ("Cmds"=w291:string[])  [unwired: 10 in]
                n89 = Build Array (concatenate)(w291, string[] ["p", "x", "X"]) -> (w290:string[])
                n90 = Not(x=w281) -> (.not. x?=w280:bool)
                n91 = for {
                  tunnel: [w300] -> w287
                  shift-right: [w301] -> w293
                  shift-left: w294 -> [w302]
                  tunnel: w290 -> [w299] mode=indexing
                  tunnel: [w298] -> w276
                  n92 = call "Mark10 Comm.vi"("Action"=Mark10_Comm_states."Write Data", "error in (no error)"=w302, "Write"=w299) -> ("error out"=w301:errorcluster, "Flags"=w300:T15, "Load"=w298:dbl)  [unwired: 2 in, 4 out]
                }
                n93 = Unbundle By Name(w287) -> ("Stopped"=w288:bool)
                n94 = Greater Or Equal?(x=w276, y=0.2) -> (x >= y?=w283:bool)
                n95 = Bundle By Name(cluster=w278, "Live Load"=w276) -> (w277:T18)
                n96 = And(x=w280, y=w283) -> (x .and. y?=w282:bool)
                n97 = Or(x=w282, y=w288) -> (x .or. y?=w286:bool)
              }
              frame True {
              }
            }
            n98 = case shown="거짓" w262 {
              tunnel: w264 -> [w272 w275]
              tunnel: [w272 w274] -> w263
              tunnel: [w271 w273] -> w261
              tunnel: w260 -> [w271 _]
              frame False {
              }
              frame True {
                n99 = call "StopMotor.vi"("error in (no error)"=w275) -> ("error out"=w274:errorcluster, "Stopped"=w273:bool)  [unwired: 9 in]
              }
            }
          }
          frame "Goto Device Surface" {
            n100 = Unbundle By Name(w308) -> ("DevFound?"=w307:bool)
            n101 = case shown="거짓" w307 {
              tunnel: w308 -> [w317 w363]
              tunnel: [w332 w365] -> w311
              tunnel: [w334 w357] -> w310
              tunnel: [_ w359] -> w309
              frame False {
                n102 = Unbundle By Name(w317) -> ("Mark10 Config.H2S%"=w312:dbl[], "Mark10 Config.H2S Speed"=w313:dbl[], "Mark10 Config.H to S"=w314:dbl)
                n103 = call "Mark10 Comm.vi"("Action"=Mark10_Comm_states."Write Data", "Write"="x" ("element")) -> ("error out"=w336:errorcluster, "Position"=w315:dbl)  [unwired: 3 in, 5 out]
                n104 = call "Mark10 Speed Calc.vi"("Home to Surface"=w314, "Live Position"=w315, "H2S Speed"=w313, "H2S %"=w312) -> ("Speed Output"=w316:dbl)  [unwired: 7 in]
                n105 = Bundle By Name(cluster=w317, "Live Position"=w315) -> (w330:T18)
                n106 = call "GetSpeedCmd.vi"("Speed"=w316) -> ("Cmds"=w329:string[])  [unwired: 10 in]
                n107 = Build Array (concatenate)(w329, "p", "X" ("element"), "x" ("element")) -> (w326:string[])
                n108 = for {
                  tunnel: [w342] -> w323
                  shift-right: [w343] -> w335
                  shift-left: w336 -> [w344]
                  tunnel: w326 -> [w341] mode=indexing
                  tunnel: [w340] -> w319
                  tunnel: [w339] -> w318
                  n109 = call "Mark10 Comm.vi"("Action"=Mark10_Comm_states."Write Data", "error in (no error)"=w344, "Write"=w341) -> ("error out"=w343:errorcluster, "Flags"=w342:T15, "Position"=w339:dbl, "Load"=w340:dbl)  [unwired: 2 in, 3 out]
                }
                n110 = Unbundle By Name(w323) -> ("Stopped"=w324:bool)
                n111 = Greater Or Equal?(x=w319, y=0.2) -> (x >= y?=w320:bool)
                n112 = Add(x=w318, y=0.005) -> (x+y=w331:dbl)
                n113 = Or(x=w320, y=w324) -> (x .or. y?=w333:bool)
                n114 = Bundle By Name(cluster=w330, "Live Load"=w319, "Live Position"=w318, "DevPosition"=w331, "DevFound?"=w320) -> (w332:T18)
                n115 = case shown="참" w320 {
                  tunnel: w335 -> [w346 w348]
                  tunnel: [w346 w347] -> w334
                  tunnel: w333 -> [_ _]
                  frame False {
                  }
                  frame True {
                    n116 = call "StopMotor.vi"("error in (no error)"=w348) -> ("error out"=w347:errorcluster)  [unwired: 9 in, 1 out]
                  }
                }
              }
              frame True {
                n117 = Unbundle By Name(w363) -> ("DevPosition"=w362:dbl)
                n118 = for {
                  tunnel: [w377] -> w364
                  shift-right: [w378] -> w358
                  shift-left: _ -> [w379]
                  tunnel: string[] ["u", "e0.10", "x", "X", "p"] -> [w376] mode=indexing
                  tunnel: [w375] -> w350
                  tunnel: [w374] -> w349
                  n119 = call "Mark10 Comm.vi"("Action"=Mark10_Comm_states."Write Data", "error in (no error)"=w379, "Write"=w376) -> ("error out"=w378:errorcluster, "Flags"=w377:T15, "Position"=w375:dbl, "Load"=w374:dbl)  [unwired: 2 in, 3 out]
                }
                n120 = Less Or Equal?(x=w362, y=w350) -> (x <= y?=w353:bool)
                n121 = Unbundle By Name(w364) -> ("Stopped"=w361:bool)
                n122 = Less Or Equal?(x=w349, y=0.2) -> (x <= y?=w352:bool)
                n123 = And(x=w353, y=w352) -> (x .and. y?=w355:bool)
                n124 = Compound Arithmetic op=AND(w353, invert w352) -> (w351:bool)
                n125 = Or(x=w355, y=w361) -> (x .or. y?=w359:bool)
                n126 = case shown="거짓" w351 {
                  tunnel: w363 -> [w369 w370]
                  tunnel: [w368 w370] -> w354
                  tunnel: w350 -> [w367 _]
                  frame False {
                    n127 = Bundle By Name(cluster=w369, "DevPosition"=w367) -> (w368:T18)
                  }
                  frame True {
                  }
                }
                n128 = Not(x=w359) -> (.not. x?=w360:bool)
                n129 = case shown="참" w359 {
                  tunnel: w358 -> [w371 w373]
                  tunnel: [w371 w372] -> w357
                  frame False {
                  }
                  frame True {
                    n130 = call "StopMotor.vi"("error in (no error)"=w373) -> ("error out"=w372:errorcluster)  [unwired: 9 in, 1 out]
                  }
                }
                n131 = Bundle By Name(cluster=w354, "Live Load"=w349, "Live Position"=w350, "DevFound?"=w360) -> (w365:T18)
              }
            }
          }
          frame "Stop Motor", Default {
            n132 = call "StopMotor.vi"("error in (no error)"=errorcluster {"status"=FALSE, "code"=0, "source"=""}) -> ("error out"=w385:errorcluster, "Stopped"=w384:bool)  [unwired: 9 in]
            n133 = Bundle By Name(cluster=w386, "Counter"=0) -> (w383:T18)
          }
          frame "Shutdown" {
          }
          frame "Exit" {
            n134 = call "Mark10 Comm.vi"("Action"=Mark10_Comm_states."Close Session") -> ("error out"=w388:errorcluster)  [unwired: 4 in, 6 out]
          }
        }
      }
      n135 = Unbundle By Name(w14) -> ("Live Load"=→"Live Load":dbl, "Live Position"=→"Live Position":dbl, "Flags"=→"Flags":T15)
    }
  }
  "error out" <- w4
  "Done?" <- w3
